vi "Read latest honor.vi"(8 "error in (no error)":errorcluster, 11 "Bobby Jones in":refnum<class "Bobby Jones.lvclass">) -> (0 "error out":errorcluster, 2 "latest honor":string, 3 "Bobby Jones out":refnum<class "Bobby Jones.lvclass">)   [LabVIEW 2019, in "Bobby Jones.lvclass"]
uses:
  Bobby Jones.lvclass
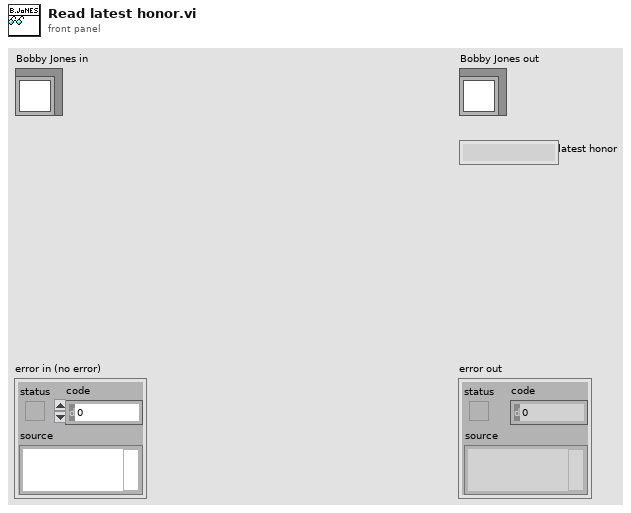
[diagram p1: front panel]
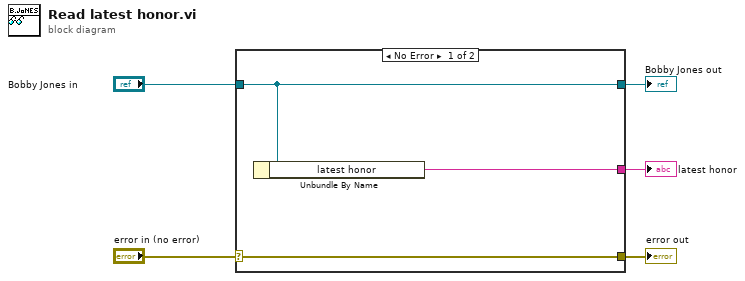
[diagram p0: block diagram]
diagram:
  n1 = case shown="No Error" "error in (no error)" {
    selector: "error in (no error)" -> [w8 w9]
    tunnel: [w8 w9] -> w4
    tunnel: [w7 w10] -> w2
    tunnel: "Bobby Jones in" -> [w7 w10]
    tunnel: [w6 _] -> w1
    frame No Error {
      n2 = Unbundle By Name(w7) -> ("latest honor"=w6:string)
    }
    frame Error {
    }
  }
  "error out" <- w4
  "Bobby Jones out" <- w2
  "latest honor" <- w1
